vi "Browse VI Ref.vi"(8 "error in (no error)":errorcluster, 10 "References":T1) -> (0 "error out":errorcluster, 2 "Name":string)   [LabVIEW 2014, in "UI Reference editor node.lvclass"]
uses:
  UI Reference editor node.lvclass
  <vilib>/NI/DCAF/Tag Editor Core/Table API/Table Manager/object ref.ctl
  <vilib>/NI/DCAF/Tag Editor Core/Configuration Editor/Classes/Engine Parent/Engine Parent Editor Node.lvclass
  <vilib>/NI/DCAF/Tag Editor Core/Configuration Editor/Classes/Module editor node/module editor node.lvclass
  module/configuration/UI Reference configuration.lvclass
  <vilib>/NI/DCAF/Tag Editor Core/Table API/Table Manager/Table Manager.lvclass
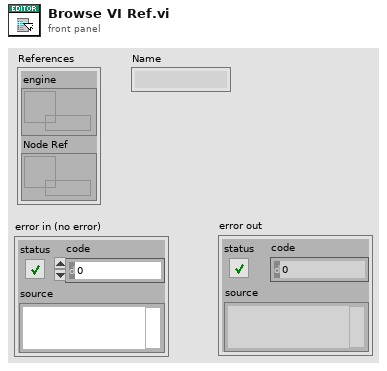
[diagram p1: front panel]
types:
  T1 = typedef "Table Manager.lvlib/Table Manager.lvclass/object ref.ctl" = cluster{"engine":refnum<data-value>, "Node Ref":refnum<data-value>}
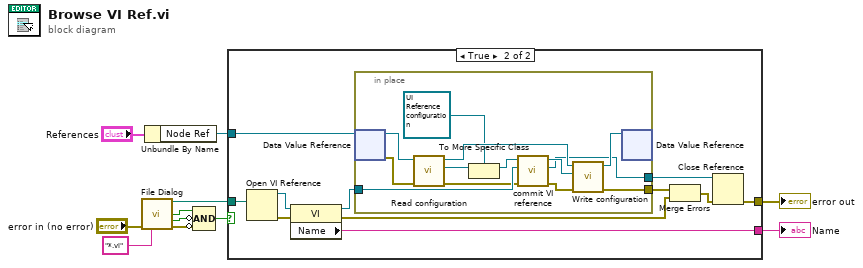
[diagram p0: block diagram]
diagram:
  n1 = call "File Dialog"("error in"="error in (no error)", "pattern (all files)"="*.vi") -> ("selected path"=w6:path, "exists"=w9:bool, "cancelled"=w10:bool, "error out"=w11:errorcluster)  [unwired: 10 in]
  n2 = Unbundle By Name("References") -> ("Node Ref"=w3:refnum<data-value>)
  n3 = Compound Arithmetic op=AND(w9, invert w10, invert w11) -> (w7:bool)
  n4 = case shown="True" w7 {
    tunnel: w6 -> [_ w22]
    tunnel: [_ w20] -> w4
    tunnel: w3 -> [_ w19]
    tunnel: [_ w13] -> w1
    frame False {
    }
    frame True {
      n5 = Open VI Reference(vi path=w22) -> (vi reference=w21:refnum<vi>, error out=w17:errorcluster)  [unwired: 5 in]
      n6 = property class="VI"(reference=w21, error in=w17) -> (reference out=w18:refnum<vi>, error out=w15:errorcluster, "Name"=w20:string)
      n7 = in-place {
        in-place-border: w18 -> [w32]
        in-place-border: [w24] -> w16
        in-place-border: [w23] -> w12
        n8 = in-place-dvr #1(w19) -> (w31:refnum<class "module editor node.lvclass">, w27:errorcluster)
        n9 = call-dynamic "Read configuration.vi"("error in"=w27, "NISE_CEF_serializable node in"=w31) -> ("error out"=w26:errorcluster, "configuration"=w30:refnum<class "NISE_CEF_serializable configuration.lvclass">, "NISE_CEF_serializable node out"=w34:refnum<class "module editor node.lvclass">)  [unwired: 7 in]
        n10 = To More Specific Class(target class=refnum<class "UI Reference configuration.lvclass"> refnum ("UI Reference configuration"), reference=w30) -> (specific class reference=w28:refnum<class "UI Reference configuration.lvclass">)  [unwired: 1 in, 1 out]
        n11 = call "commit VI reference.vi"("error in"=w26, "VI Refnum in"=w32, "UI Reference configuration in"=w28) -> ("error out"=w25:errorcluster, "VI Refnum out"=w23:refnum<vi>, "UI Reference configuration out"=w33:refnum<class "UI Reference configuration.lvclass">)  [unwired: 6 in]
        n12 = call-dynamic "Write configuration.vi"("error in"=w25, "configuration"=w33, "NISE_CEF_serializable node in"=w34) -> ("error out"=w24:errorcluster, "NISE_CEF_serializable node out"=w35:refnum<class "module editor node.lvclass">)  [unwired: 7 in]
        n13 = in-place-dvr #1(w35) -> ()  [unwired: 2 out]
      }
      n14 = Merge Errors(w16, w15) -> (w14:errorcluster)
      n15 = Close Reference(reference=w12, error in (no error)=w14) -> (error out=w13:errorcluster)
    }
  }
  "Name" <- w4
  "error out" <- w1
